vi "to string.vi"(8 "error in":errorcluster, 11 "Simple Sequencer TBM configuration in":refnum<class "Simple Sequencer TBM configuration.lvclass">) -> (0 "error out":errorcluster, 1 "data":string, 2 "version":string, 3 "Simple Sequencer TBM configuration out":refnum<class "Simple Sequencer TBM configuration.lvclass">)   [LabVIEW 2014, in "Simple Sequencer TBM configuration.lvclass"]
doc: "Provides an interface for saving a module configuration to a file or other serialized data source. It is recommended that all children of this class store data in two sets--data required for its own initialization, and any data required for parent initialization--and that each implementation uses the <b>Call Parent Method</b> primitive to serialize parent information."
uses:
  Simple Sequencer TBM configuration.lvclass
  Simple Sequencer TBM configuration.lvclass/Simple Sequencer TBM configuration.ctl
  current version.vi
  sequencer parent classes/sequencer config parent/base TBM sequencer configuration.lvclass
  sequencer parent classes/action configuration parent/action configuration.lvclass
  <vilib>/NI/Configuration Framework/serializable configuration/NISE_CEF_serializable configuration.lvclass
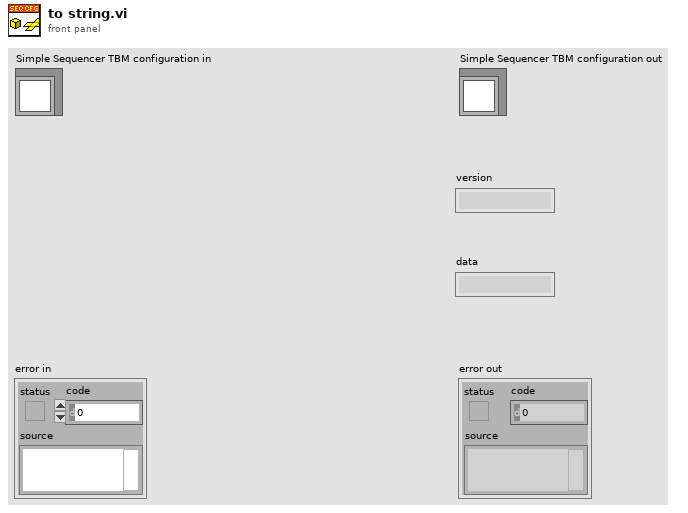
[diagram p1: front panel]
types:
  T1 = typedef "Simple Sequencer TBM configuration.lvclass/sequence definition.ctl" = cluster{"sequence name":string, "action configs":refnum<class "action configuration.lvclass">[]}
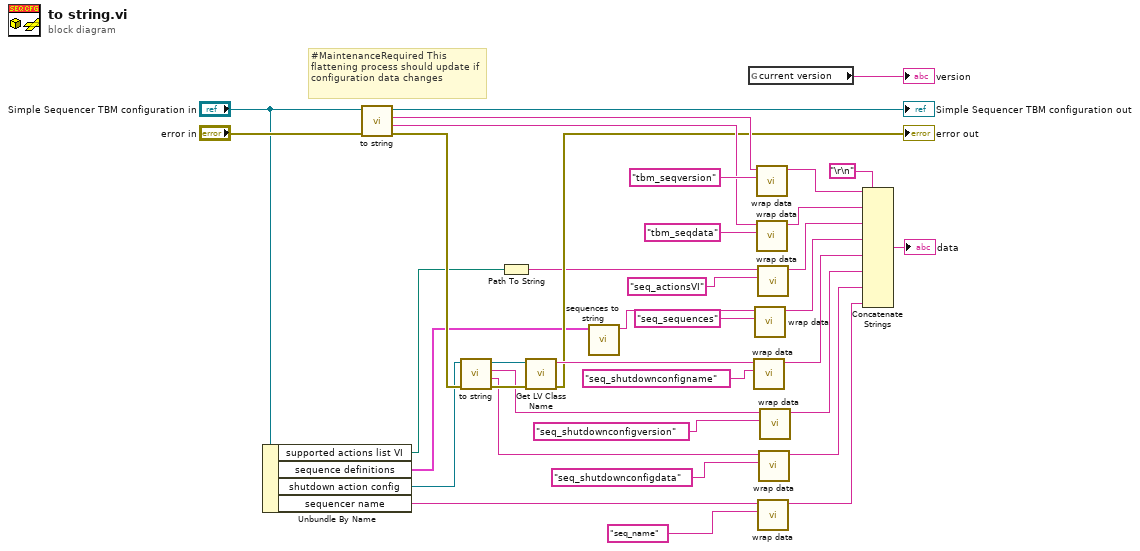
[diagram p0: block diagram]
diagram:
  w3 = "\r\n"
  # "#MaintenanceRequired This flattening process should update if configuration data changes"
  n1 = Unbundle By Name("Simple Sequencer TBM configuration in") -> ("supported actions list VI"=w2:path, "sequence definitions"=w8:T1[], "shutdown action config"=w6:refnum<class "action configuration.lvclass">, "sequencer name"=w21:string)
  n2 = call-parent "to string.vi"("error in"="error in", "engine configuration in"="Simple Sequencer TBM configuration in") -> ("error out"=w15:errorcluster, "data"=w29:string, "version"=w30:string, "engine configuration out"=→"Simple Sequencer TBM configuration out":refnum<class "Simple Sequencer TBM configuration.lvclass">)  [unwired: 6 in]
  n3 = call-dynamic "to string.vi"("error in"=w15, "configuration in"=w6) -> ("error out"=w14:errorcluster, "data"=w11:string, "version"=w12:string, "configuration out"=w16:refnum<class "action configuration.lvclass">)  [unwired: 6 in]
  n4 = Path To String(path=w2) -> (string=w1:string)
  n5 = call <vilib>:"Get LV Class Name.vi"("error in (no error)"=w14, "object"=w16) -> ("error out"=→"error out":errorcluster, "class name"=w19:string)  [unwired: 8 in]
  n6 = call "sequences to string.vi"("sequence definitions"=w8) -> ("string"=w7:string)  [unwired: 10 in]
  n7 = global read "current version.vi" "current version"() -> (→"version":string)
  n8 = call <vilib>:"wrap data.vi"("identifier"="seq_shutdownconfigname", "data to wrap"=w19) -> ("wrapped data"=w10:string)  [unwired: 9 in]
  n9 = call <vilib>:"wrap data.vi"("identifier"="seq_sequences", "data to wrap"=w7) -> ("wrapped data"=w24:string)  [unwired: 9 in]
  n10 = call <vilib>:"wrap data.vi"("identifier"="tbm_seqversion" ("additional identifier"), "data to wrap"=w30) -> ("wrapped data"=w32:string)  [unwired: 9 in]
  n11 = call <vilib>:"wrap data.vi"("identifier"="tbm_seqdata" ("additional identifier"), "data to wrap"=w29) -> ("wrapped data"=w31:string)  [unwired: 9 in]
  n12 = call <vilib>:"wrap data.vi"("identifier"="seq_actionsVI", "data to wrap"=w1) -> ("wrapped data"=w4:string)  [unwired: 9 in]
  n13 = call <vilib>:"wrap data.vi"("identifier"="seq_name", "data to wrap"=w21) -> ("wrapped data"=w20:string)  [unwired: 9 in]
  n14 = call <vilib>:"wrap data.vi"("identifier"="seq_shutdownconfigdata", "data to wrap"=w11) -> ("wrapped data"=w23:string)  [unwired: 9 in]
  n15 = call <vilib>:"wrap data.vi"("identifier"="seq_shutdownconfigversion", "data to wrap"=w12) -> ("wrapped data"=w9:string)  [unwired: 9 in]
  n16 = Concatenate Strings(w32, w3, w31, w3, w4, w3, w24, w3, w10, w3, w9, w3, w23, w3, w20) -> (→"data":string)
